vi "filter.debug.vi"(11 "filter.data in":T1 {"get.state"."v"."Quantity" format="%.0x"; "get.state"."v"."OrderId" format="%.0x"; "mem.cmd"."ord.2"."v"."Quantity" format="%016x"; "mem.cmd"."ord.2"."v"."OrderId" format="%016x"; "mem.cmd"."ord.1"."v"."Quantity" format="%016x"; "mem.cmd"."ord.1"."v"."OrderId" format="%016x"; "mem.cmd"."ticker"."v"."Symbol" format="%016x"; "mem.cmd"."order.slot.value"."Quantity" format="%016x"; "mem.cmd"."order.slot.value"."OrderId" format="%016x"; "debug"."v"."slot.3" format="%.0x"; "debug"."v"."slot.2" format="%.0x"; "debug"."v"."slot.1" format="%.0x"; "debug"."v"."slot.0" format="%.0x"; "Scratch"."OrderId" format="%016x"; "hash.2"."data.in" format="%.0x"; "hash.2"."crc32.out" format="%.0x"; "hash.1"."data.in" format="%.0x"; "hash.1"."crc32.out" format="%.0x"}) -> (3 "filter.data out":T1 {"get.state"."v"."Quantity" format="%.0x"; "get.state"."v"."OrderId" format="%.0x"; "mem.cmd"."ord.2"."v"."Quantity" format="%016x"; "mem.cmd"."ord.2"."v"."OrderId" format="%016x"; "mem.cmd"."ord.1"."v"."Quantity" format="%016x"; "mem.cmd"."ord.1"."v"."OrderId" format="%016x"; "mem.cmd"."ticker"."v"."Symbol" format="%016x"; "mem.cmd"."order.slot.value"."Quantity" format="%016x"; "mem.cmd"."order.slot.value"."OrderId" format="%016x"; "debug"."v"."slot.3" format="%.0x"; "debug"."v"."slot.2" format="%.0x"; "debug"."v"."slot.1" format="%.0x"; "debug"."v"."slot.0" format="%.0x"; "Scratch"."OrderId" format="%016x"; "hash.2"."data.in" format="%.0x"; "hash.2"."crc32.out" format="%.0x"; "hash.1"."data.in" format="%.0x"; "hash.1"."crc32.out" format="%.0x"})   [LabVIEW 2020]
uses:
  order.slot.ctl
  ticker.slot.ctl
  filter.memory.command.ctl
  filter.debug.slot.ctl
  filter.debug.ctl
  filter.states.ctl
  order.slot.hm.ctl
  order.slot.access.ctl
  ticker.slot.access.ctl
  filter.data.scratch.ctl
  Market.Data.Common/fpga/orderbook.command.ctl
  Market.Data.Common/fpga/fpganow.common.fpga.lvlib
  filter.data.ctl
  filter.state.slot.ctl
  filter.state.ctl
  Market.Data.Common/fpga/orderbook.command.type.ctl
  filter.hash.ctl
  Filter.lvclass
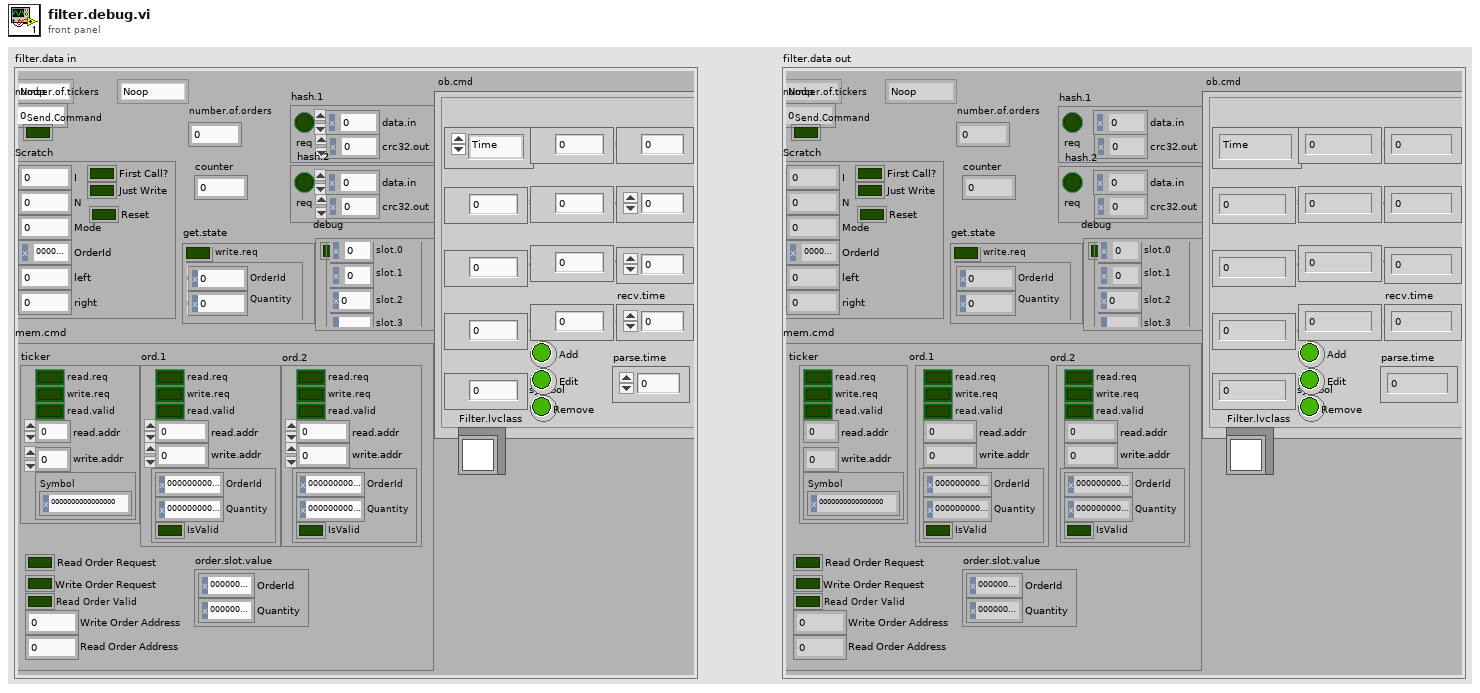
[diagram p1: front panel]
types:
  T1 = typedef "filter.data.ctl" = cluster{"filter.state":T2, "number.of.tickers":u32, "filter.saved.state":T2, "Send.Command":bool, "hash.1":T3, "hash.2":T3, "Scratch":T4, "debug":T5, "mem.cmd":T7, "get.state":T13, "ob.cmd":T15, "number.of.orders":u32, "Filter.lvclass":refnum<class "Filter.lvclass">, "counter":i16}
  T2 = typedef "filter.states.ctl" = enum16{"Noop", "Reset", "Debug", "Configuration", "Wait.for.Command", "Filter.Add", "Filter.Other", "Insert.Order", "Delete Order", "Get.State", "Get.Watchlist", "Get.Memory"}
  T3 = typedef "filter.hash.ctl" = cluster{"req":bool, "data.in":u64, "crc32.out":u32}
  T4 = typedef "filter.data.scratch.ctl" = cluster{"I":u32, "N":u32, "Mode":u32, "OrderId":u64, "First Call?":bool, "Just Write":bool, "left":u32, "right":u32, "Reset":bool}
  T5 = typedef "filter.debug.ctl" = cluster{"write":bool, "v":T6}
  T6 = typedef "filter.debug.slot.ctl" = cluster{"slot.0":u64, "slot.1":u64, "slot.2":u64, "slot.3":u64}
  T7 = typedef "filter.memory.command.ctl" = cluster{"Read Order Request":bool, "Write Order Request":bool, "Read Order Valid":bool, "Write Order Address":u32, "Read Order Address":u32, "order.slot.value":T8, "ticker":T9, "ord.1":T11, "ord.2":T11}
  T8 = typedef "order.slot.ctl" = cluster{"OrderId":u64, "Quantity":u64}
  T9 = typedef "ticker.slot.access.ctl" = cluster{"read.req":bool, "write.req":bool, "read.valid":bool, "read.addr":u32, "write.addr":u32, "v":T10}
  T10 = typedef "ticker.slot.ctl" = cluster{"Symbol":u64}
  T11 = typedef "order.slot.access.ctl" = cluster{"read.req":bool, "write.req":bool, "read.valid":bool, "read.addr":u32, "write.addr":u32, "v":T12}
  T12 = typedef "order.slot.hm.ctl" = cluster{"OrderId":u64, "Quantity":u64, "IsValid":bool}
  T13 = typedef "filter.state.ctl" = cluster{"write.req":bool, "v":T14}
  T14 = typedef "filter.state.slot.ctl" = cluster{"OrderId":u64, "Quantity":u64}
  T15 = typedef "fpganow.common.fpga.lvlib/orderbook.command.ctl" = cluster{"type":T16, "side":u8, "orderId ":u64, "quantity":u32, "symbol":u64, "price":u64, "executed.qty":u32, "canceled.qty":u32, "remaining.qty":u32, "seconds":u64, "nanoseconds":u64, "Add":bool, "Edit":bool, "Remove":bool, "seq no":u32, "recv.time":u64, "parse.time":u64}
  T16 = typedef "fpganow.common.fpga.lvlib/orderbook.command.type.ctl" = enum8{"Time", "AddOrder", "OrderExecuted", "OrderExecutedAtPrice", "ReduceSize", "ModifyOrder", "DeleteOrder", "Get.Everything", "Get.All.Orders", "Get.Top"}
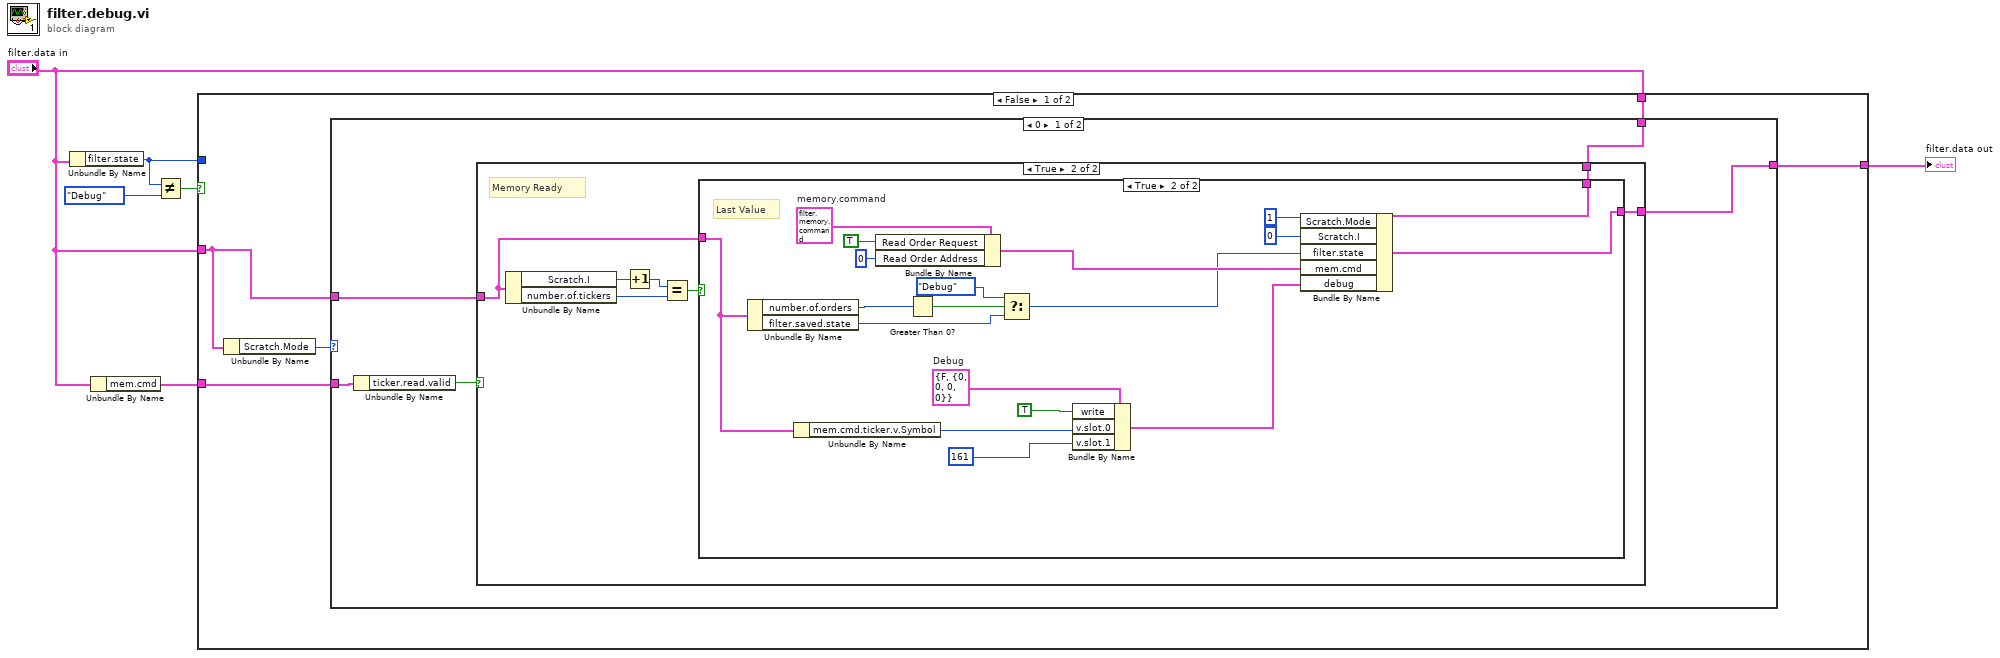
[diagram p0: block diagram]
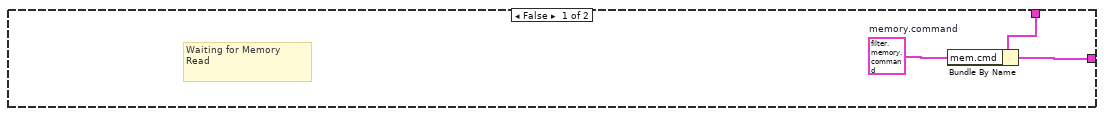
[diagram p2: hidden frame]
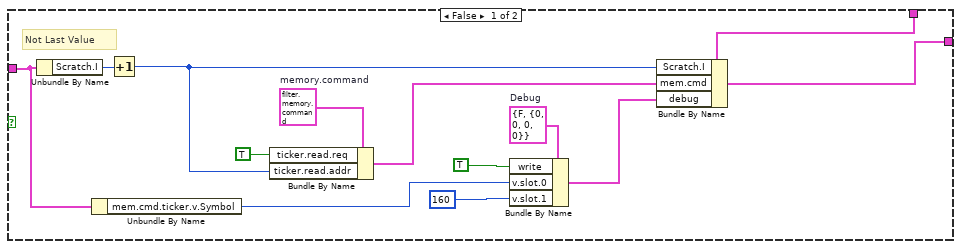
[diagram p3: hidden frame]
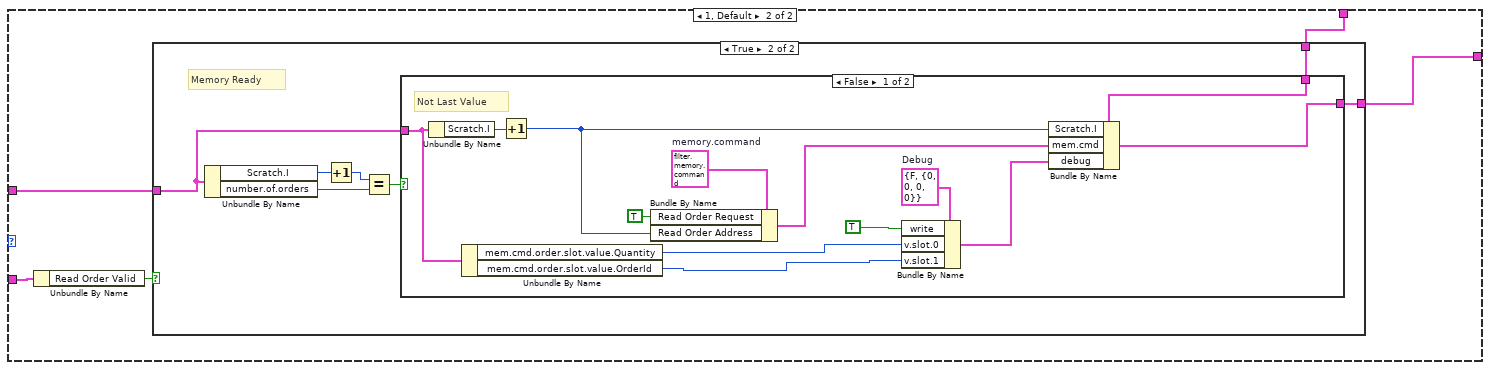
[diagram p4: hidden frame]
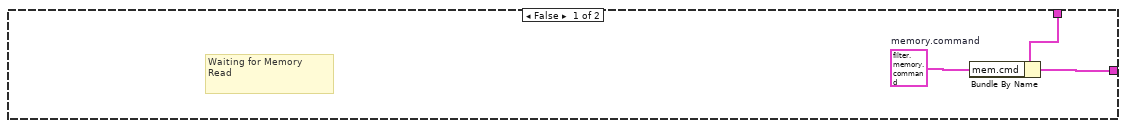
[diagram p5: hidden frame]
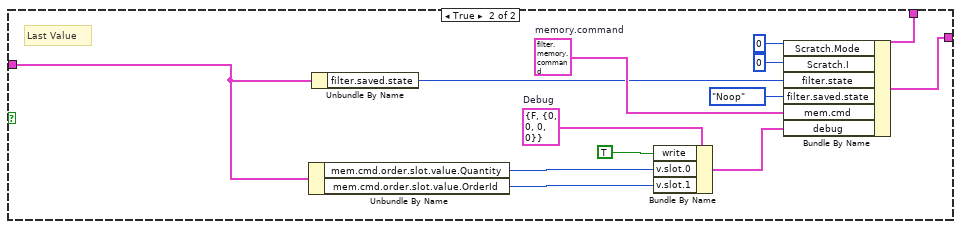
[diagram p6: hidden frame]
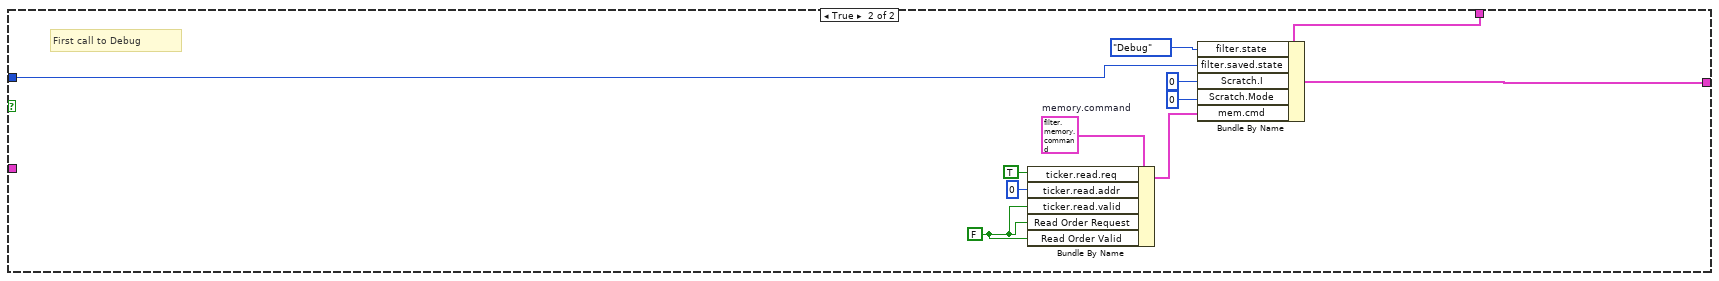
[diagram p7: hidden frame]
diagram:
  n1 = Unbundle By Name("filter.data in") -> ("filter.state"=w3:T2)
  n2 = Unbundle By Name("filter.data in") -> ("mem.cmd"=w5:T7)
  n3 = Not Equal?(x=w3, y=filter.states."Debug" ("filter.state")) -> (x != y?=w2:bool)
  n4 = case shown="False" w2 {
    tunnel: "filter.data in" -> [w10 w110]
    tunnel: [w11 w109] -> w1
    tunnel: w3 -> [_ w107]
    tunnel: "filter.data in" -> [w8 _]
    tunnel: w5 -> [w9 _]
    frame False {
      n5 = Unbundle By Name(w8) -> ("Scratch.Mode"=w7:u32)
      n6 = case shown="0" w7 {
        tunnel: [w16 w63] -> w11
        tunnel: w10 -> [w15 w62]
        tunnel: w9 -> [w13 w60]
        tunnel: w8 -> [w12 w59]
        frame 0 {
          n7 = Unbundle By Name(w13) -> ("ticker.read.valid"=w14:bool)
          n8 = case shown="True" w14 {
            tunnel: [w17 w20] -> w16
            tunnel: w15 -> [w19 w21]
            tunnel: w12 -> [_ w22]
            frame False {
              w18 = T7 {"Read Order Request"=FALSE, "Write Order Request"=FALSE, "Read Order Valid"=FALSE, "Write Order Address"=0, "Read Order Address"=0, "order.slot.value"={"OrderId"=0, "Quantity"=0}, "ticker"={"read.req"=FALSE, "write.req"=FALSE, "read.valid"=FALSE, "read.addr"=0, "write.addr"=0, "v"={"Symbol"=0}}, "ord.1"={"read.req"=FALSE, "write.req"=FALSE, "read.valid"=FALSE, "read.addr"=0, "write.addr"=0, "v"={"OrderId"=0, "Quantity"=0, "IsValid"=FALSE}}, "ord.2"={"read.req"=FALSE, "write.req"=FALSE, "read.valid"=FALSE, "read.addr"=0, "write.addr"=0, "v"={"OrderId"=0, "Quantity"=0, "IsValid"=FALSE}}}  # memory.command
              # "Waiting for Memory\nRead"
              n9 = Bundle By Name(cluster=w19, "mem.cmd"=w18) -> (w17:T1)
            }
            frame True {
              # "Memory Ready"
              n10 = Unbundle By Name(w22) -> ("Scratch.I"=w26:u32, "number.of.tickers"=w24:u32)
              n11 = Increment(x=w26) -> (x+1=w25:u32)
              n12 = Equal?(x=w25, y=w24) -> (x = y?=w23:bool)
              n13 = case shown="True" w23 {
                tunnel: w22 -> [w32 w45]
                tunnel: w21 -> [w28 w58]
                tunnel: [w39 w57] -> w20
                frame False {
                  w35 = T5 {"write"=FALSE, "v"={"slot.0"=0, "slot.1"=0, "slot.2"=0, "slot.3"=0}}  # Debug
                  w38 = T7 {"Read Order Request"=FALSE, "Write Order Request"=FALSE, "Read Order Valid"=FALSE, "Write Order Address"=0, "Read Order Address"=0, "order.slot.value"={"OrderId"=0, "Quantity"=0}, "ticker"={"read.req"=FALSE, "write.req"=FALSE, "read.valid"=FALSE, "read.addr"=0, "write.addr"=0, "v"={"Symbol"=0}}, "ord.1"={"read.req"=FALSE, "write.req"=FALSE, "read.valid"=FALSE, "read.addr"=0, "write.addr"=0, "v"={"OrderId"=0, "Quantity"=0, "IsValid"=FALSE}}, "ord.2"={"read.req"=FALSE, "write.req"=FALSE, "read.valid"=FALSE, "read.addr"=0, "write.addr"=0, "v"={"OrderId"=0, "Quantity"=0, "IsValid"=FALSE}}}  # memory.command
                  # "Not Last Value"
                  n14 = Unbundle By Name(w32) -> ("Scratch.I"=w36:u32)
                  n15 = Unbundle By Name(w32) -> ("mem.cmd.ticker.v.Symbol"=w31:u64)
                  n16 = Increment(x=w36) -> (x+1=w29:u32)
                  n17 = Bundle By Name(cluster=w38, "ticker.read.req"=TRUE ("Read.Request"), "ticker.read.addr"=w29) -> (w37:T7)
                  n18 = Bundle By Name(cluster=w35, "write"=TRUE ("Write.to.Debug"), "v.slot.0"=w31, "v.slot.1"=u64 160 ("debug.slot.OrderId")) -> (w34:T5)
                  n19 = Bundle By Name(cluster=w28, "Scratch.I"=w29, "mem.cmd"=w37, "debug"=w34) -> (w39:T1)
                }
                frame True {
                  w56 = T5 {"write"=FALSE, "v"={"slot.0"=0, "slot.1"=0, "slot.2"=0, "slot.3"=0}}  # Debug
                  w49 = T7 {"Read Order Request"=FALSE, "Write Order Request"=FALSE, "Read Order Valid"=FALSE, "Write Order Address"=0, "Read Order Address"=0, "order.slot.value"={"OrderId"=0, "Quantity"=0}, "ticker"={"read.req"=FALSE, "write.req"=FALSE, "read.valid"=FALSE, "read.addr"=0, "write.addr"=0, "v"={"Symbol"=0}}, "ord.1"={"read.req"=FALSE, "write.req"=FALSE, "read.valid"=FALSE, "read.addr"=0, "write.addr"=0, "v"={"OrderId"=0, "Quantity"=0, "IsValid"=FALSE}}, "ord.2"={"read.req"=FALSE, "write.req"=FALSE, "read.valid"=FALSE, "read.addr"=0, "write.addr"=0, "v"={"OrderId"=0, "Quantity"=0, "IsValid"=FALSE}}}  # memory.command
                  # "Last Value"
                  n20 = Unbundle By Name(w45) -> ("number.of.orders"=w44:u32, "filter.saved.state"=w40:T2)
                  n21 = Unbundle By Name(w45) -> ("mem.cmd.ticker.v.Symbol"=w53:u64)
                  n22 = Bundle By Name(cluster=w49, "Read Order Request"=TRUE ("Read Order\nRequest"), "Read Order Address"=u32 0 ("Read Order\nAddress")) -> (w48:T7)
                  n23 = Greater Than 0?(x=w44) -> (x > 0?=w43:bool)
                  n24 = Select(t=filter.states."Debug" ("filter.state"), s=w43, f=w40) -> (s? t:f=w41:T2)
                  n25 = Bundle By Name(cluster=w56, "write"=TRUE ("Write.to.Debug"), "v.slot.0"=w53, "v.slot.1"=u64 161 ("debug.slot.OrderId")) -> (w55:T5)
                  n26 = Bundle By Name(cluster=w58, "Scratch.Mode"=u32 1, "Scratch.I"=u32 0, "filter.state"=w41, "mem.cmd"=w48, "debug"=w55) -> (w57:T1)
                }
              }
            }
          }
        }
        frame 1, Default {
          n27 = Unbundle By Name(w60) -> ("Read Order Valid"=w61:bool)
          n28 = case shown="True" w61 {
            tunnel: [w64 w67] -> w63
            tunnel: w62 -> [w66 w68]
            tunnel: w59 -> [_ w69]
            frame False {
              w65 = T7 {"Read Order Request"=FALSE, "Write Order Request"=FALSE, "Read Order Valid"=FALSE, "Write Order Address"=0, "Read Order Address"=0, "order.slot.value"={"OrderId"=0, "Quantity"=0}, "ticker"={"read.req"=FALSE, "write.req"=FALSE, "read.valid"=FALSE, "read.addr"=0, "write.addr"=0, "v"={"Symbol"=0}}, "ord.1"={"read.req"=FALSE, "write.req"=FALSE, "read.valid"=FALSE, "read.addr"=0, "write.addr"=0, "v"={"OrderId"=0, "Quantity"=0, "IsValid"=FALSE}}, "ord.2"={"read.req"=FALSE, "write.req"=FALSE, "read.valid"=FALSE, "read.addr"=0, "write.addr"=0, "v"={"OrderId"=0, "Quantity"=0, "IsValid"=FALSE}}}  # memory.command
              # "Waiting for Memory\nRead"
              n29 = Bundle By Name(cluster=w66, "mem.cmd"=w65) -> (w64:T1)
            }
            frame True {
              # "Memory Ready"
              n30 = Unbundle By Name(w69) -> ("Scratch.I"=w73:u32, "number.of.orders"=w71:u32)
              n31 = Increment(x=w73) -> (x+1=w72:u32)
              n32 = Equal?(x=w72, y=w71) -> (x = y?=w70:bool)
              n33 = case shown="False" w70 {
                tunnel: w69 -> [w79 w94]
                tunnel: w68 -> [w77 w99]
                tunnel: [w86 w98] -> w67
                frame False {
                  w82 = T5 {"write"=FALSE, "v"={"slot.0"=0, "slot.1"=0, "slot.2"=0, "slot.3"=0}}  # Debug
                  w85 = T7 {"Read Order Request"=FALSE, "Write Order Request"=FALSE, "Read Order Valid"=FALSE, "Write Order Address"=0, "Read Order Address"=0, "order.slot.value"={"OrderId"=0, "Quantity"=0}, "ticker"={"read.req"=FALSE, "write.req"=FALSE, "read.valid"=FALSE, "read.addr"=0, "write.addr"=0, "v"={"Symbol"=0}}, "ord.1"={"read.req"=FALSE, "write.req"=FALSE, "read.valid"=FALSE, "read.addr"=0, "write.addr"=0, "v"={"OrderId"=0, "Quantity"=0, "IsValid"=FALSE}}, "ord.2"={"read.req"=FALSE, "write.req"=FALSE, "read.valid"=FALSE, "read.addr"=0, "write.addr"=0, "v"={"OrderId"=0, "Quantity"=0, "IsValid"=FALSE}}}  # memory.command
                  # "Not Last Value"
                  n34 = Unbundle By Name(w79) -> ("Scratch.I"=w83:u32)
                  n35 = Unbundle By Name(w79) -> ("mem.cmd.order.slot.value.Quantity"=w74:u64, "mem.cmd.order.slot.value.OrderId"=w75:u64)
                  n36 = Increment(x=w83) -> (x+1=w76:u32)
                  n37 = Bundle By Name(cluster=w85, "Read Order Request"=TRUE ("Read.Request"), "Read Order Address"=w76) -> (w84:T7)
                  n38 = Bundle By Name(cluster=w82, "write"=TRUE ("Write.to.Debug"), "v.slot.0"=w74, "v.slot.1"=w75) -> (w81:T5)
                  n39 = Bundle By Name(cluster=w77, "Scratch.I"=w76, "mem.cmd"=w84, "debug"=w81) -> (w86:T1)
                }
                frame True {
                  w97 = T5 {"write"=FALSE, "v"={"slot.0"=0, "slot.1"=0, "slot.2"=0, "slot.3"=0}}  # Debug
                  w93 = T7 {"Read Order Request"=FALSE, "Write Order Request"=FALSE, "Read Order Valid"=FALSE, "Write Order Address"=0, "Read Order Address"=0, "order.slot.value"={"OrderId"=0, "Quantity"=0}, "ticker"={"read.req"=FALSE, "write.req"=FALSE, "read.valid"=FALSE, "read.addr"=0, "write.addr"=0, "v"={"Symbol"=0}}, "ord.1"={"read.req"=FALSE, "write.req"=FALSE, "read.valid"=FALSE, "read.addr"=0, "write.addr"=0, "v"={"OrderId"=0, "Quantity"=0, "IsValid"=FALSE}}, "ord.2"={"read.req"=FALSE, "write.req"=FALSE, "read.valid"=FALSE, "read.addr"=0, "write.addr"=0, "v"={"OrderId"=0, "Quantity"=0, "IsValid"=FALSE}}}  # memory.command
                  # "Last Value"
                  n40 = Unbundle By Name(w94) -> ("mem.cmd.order.slot.value.Quantity"=w88:u64, "mem.cmd.order.slot.value.OrderId"=w87:u64)
                  n41 = Unbundle By Name(w94) -> ("filter.saved.state"=w92:T2)
                  n42 = Bundle By Name(cluster=w97, "write"=TRUE ("Write.to.Debug"), "v.slot.0"=w88, "v.slot.1"=w87) -> (w96:T5)
                  n43 = Bundle By Name(cluster=w99, "Scratch.Mode"=u32 0, "Scratch.I"=u32 0, "filter.state"=w92, "filter.saved.state"=filter.states."Noop", "mem.cmd"=w93, "debug"=w96) -> (w98:T1)
                }
              }
            }
          }
        }
      }
    }
    frame True {
      w101 = FALSE ("Read Ticker Valid")
      w103 = T7 {"Read Order Request"=FALSE, "Write Order Request"=FALSE, "Read Order Valid"=FALSE, "Write Order Address"=0, "Read Order Address"=0, "order.slot.value"={"OrderId"=0, "Quantity"=0}, "ticker"={"read.req"=FALSE, "write.req"=FALSE, "read.valid"=FALSE, "read.addr"=0, "write.addr"=0, "v"={"Symbol"=0}}, "ord.1"={"read.req"=FALSE, "write.req"=FALSE, "read.valid"=FALSE, "read.addr"=0, "write.addr"=0, "v"={"OrderId"=0, "Quantity"=0, "IsValid"=FALSE}}, "ord.2"={"read.req"=FALSE, "write.req"=FALSE, "read.valid"=FALSE, "read.addr"=0, "write.addr"=0, "v"={"OrderId"=0, "Quantity"=0, "IsValid"=FALSE}}}  # memory.command
      # "First call to Debug"
      n44 = Bundle By Name(cluster=w103, "ticker.read.req"=TRUE ("Read Ticker\nRequest"), "ticker.read.addr"=u32 0 ("Read Ticker\nAddress"), "ticker.read.valid"=w101, "Read Order Request"=w101, "Read Order Valid"=w101) -> (w104:T7)
      n45 = Bundle By Name(cluster=w110, "filter.state"=filter.states."Debug", "filter.saved.state"=w107, "Scratch.I"=u32 0, "Scratch.Mode"=u32 0, "mem.cmd"=w104) -> (w109:T1)
    }
  }
  "filter.data out" <- w1
